vi "SetWidth.vi"(8 "error in (no error)":errorcluster, 10 "Width":i16, 11 "Square in":refnum<class "Square.lvclass">) -> (0 "error out":errorcluster, 3 "Square out":refnum<class "Square.lvclass">)   [LabVIEW 2021, in "Picture2D.lvlib" / "Square.lvclass"]
uses:
  Square.lvclass
  Square.lvclass/Square.ctl
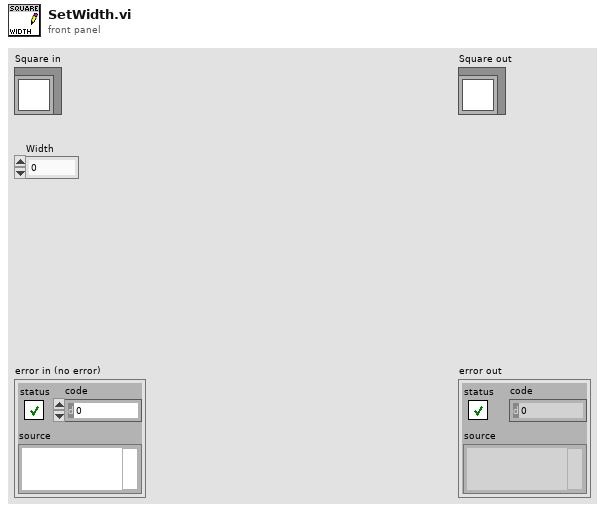
[diagram p1: front panel]
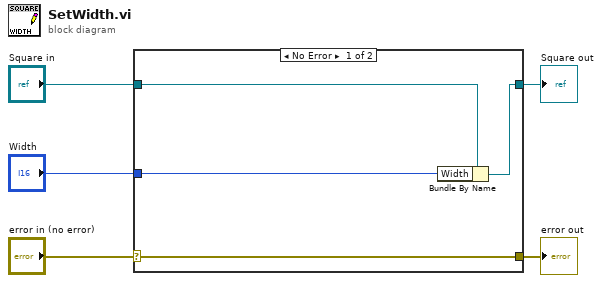
[diagram p0: block diagram]
diagram:
  n1 = case shown="No Error" "error in (no error)" {
    selector: "error in (no error)" -> [w9 w10]
    tunnel: [w9 w10] -> w4
    tunnel: [w7 w11] -> w2
    tunnel: "Square in" -> [w8 w11]
    tunnel: "Width" -> [w6 _]
    frame No Error {
      n2 = Bundle By Name(cluster=w8, "Width"=w6) -> (w7:refnum<class "Square.lvclass">)
    }
    frame Error {
    }
  }
  "error out" <- w4
  "Square out" <- w2
